vi "DMM Trig Slope.vi"(8 "error in (no error)":errorcluster, 11 "IVI Refnum in":refnum<k15>) -> (0 "error out":errorcluster, 3 "IVI Refnum out":refnum<k15>)   [LabVIEW 2019, in "SupportVIs.lvlib"]
uses:
  SupportVIs.lvlib
  <instrlib>/niDMM/nidmm.llb/niDMM Slope.ctl
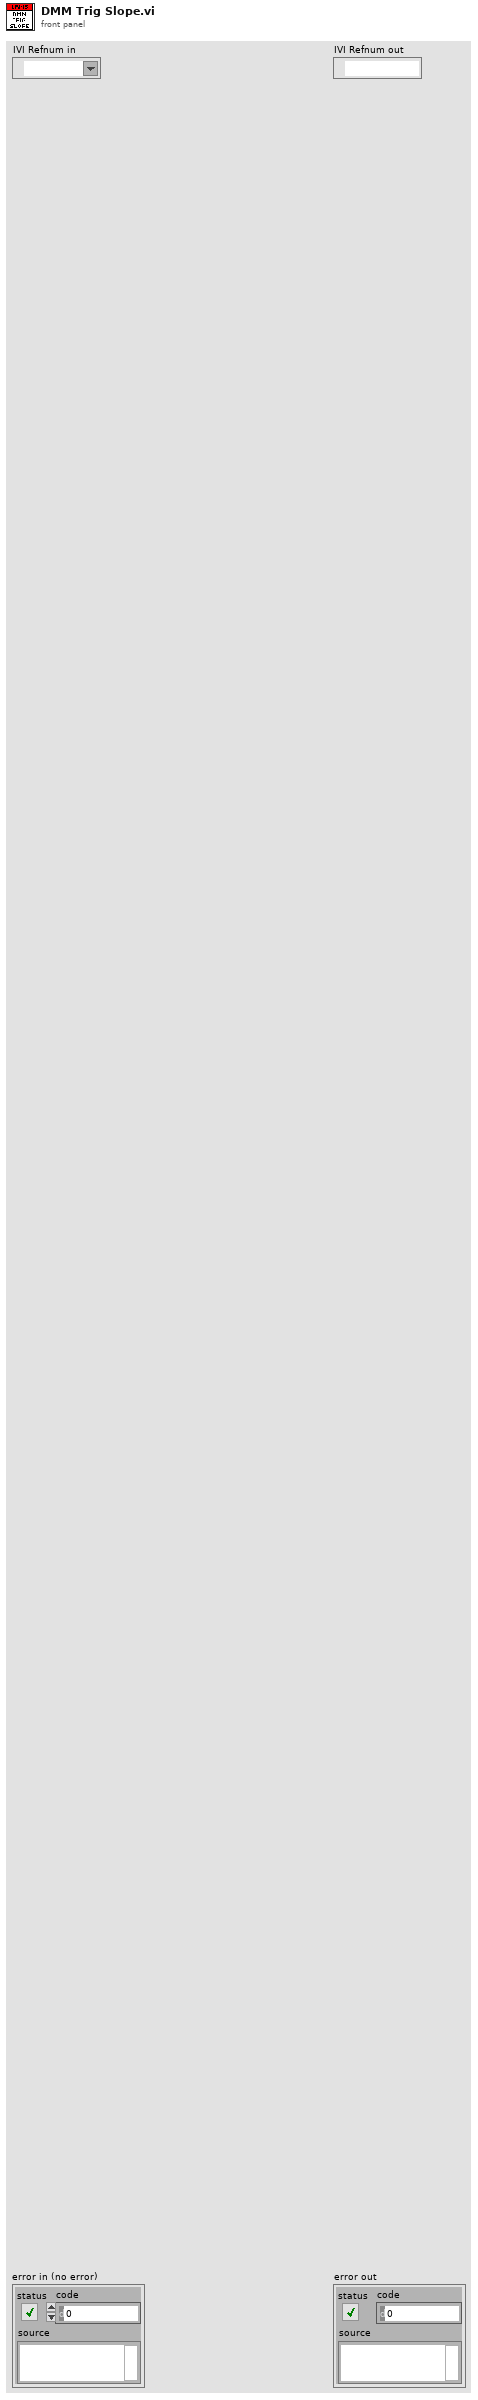
[diagram p1: front panel]
types:
  T1 = typedef "niDMM Slope.ctl" = enum16{"Rising Edge", "Falling Edge"}
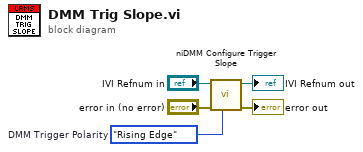
[diagram p0: block diagram]
diagram:
  w1 = niDMM_Slope."Rising Edge"  # DMM Trigger Polarity
  n1 = call <instrlib>:"niDMM Configure Trigger Slope.vi"("Slope"=w1, "error in (no error)"="error in (no error)", "instrument handle"="IVI Refnum in") -> ("error out"=→"error out":errorcluster, "instrument handle out"=→"IVI Refnum out":refnum<k15>)  [unwired: 7 in]
